vi "Read Output.vi"(8 "error in":errorcluster, 11 "2230G in":refnum<class "2230G.lvclass">) -> (0 "error out":errorcluster, 2 "Output":bool, 3 "2230G out":refnum<class "2230G.lvclass">)   [LabVIEW 2018, in "2230G.lvlib" / "2230G.lvclass"]
uses:
  2230G.lvclass
  <vilib>/regexp/Match Regular Expression.xnode
  PPLs/Power Supply/Parent/Power_Supply.lvlibp/Power Supply.lvclass
  <instrlib>/Keithley KE22xx Series/Keithley KE22xx Series.lvlib
  C:/Projects/LabVIEW/PPLs/Power Supply/Parent/Power_Supply.lvlibp/Power Supply.lvclass
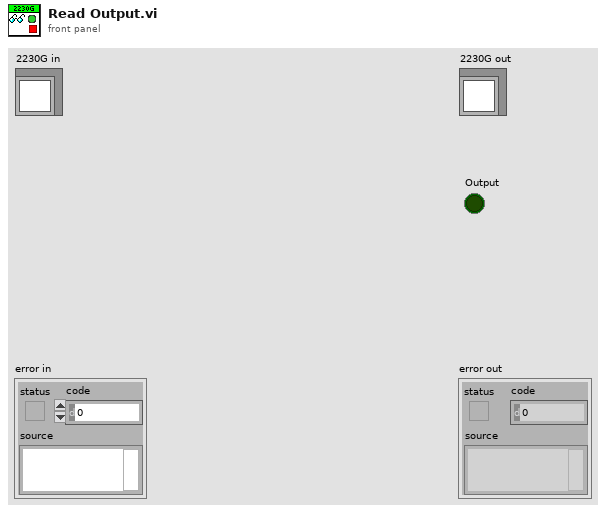
[diagram p1: front panel]
types:
  T1 = typedef "Power_Supply.lvlibp/Channel List.ctl" = enum16{"Channel 1", "Channel 2", "Channel 3", "Channel 4"}
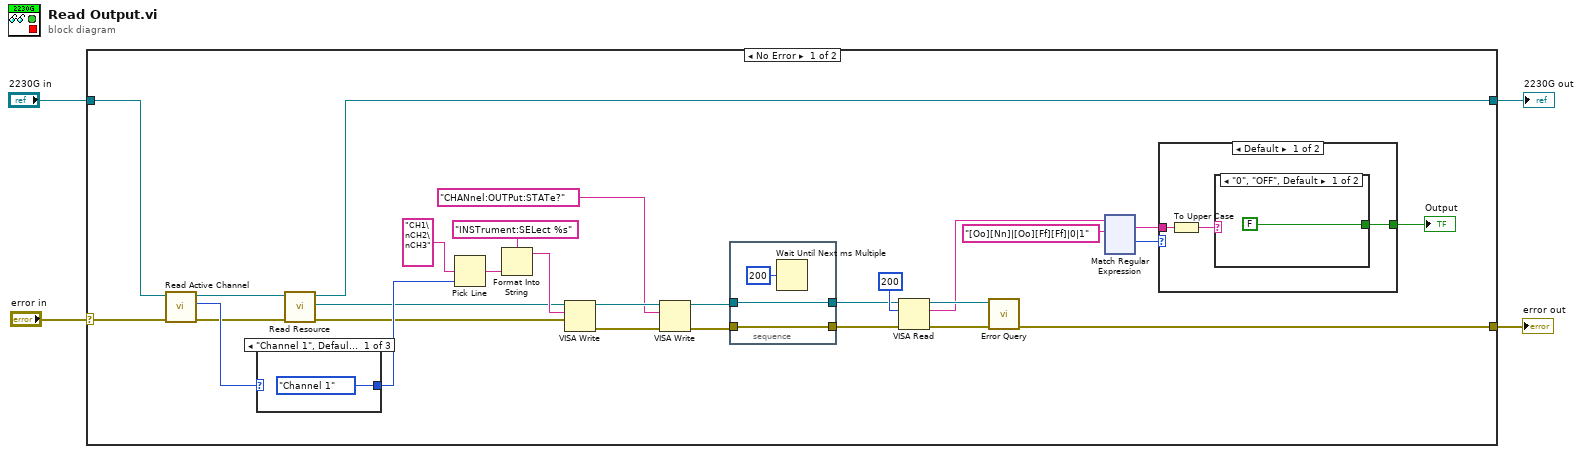
[diagram p0: block diagram]
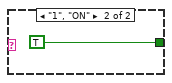
[diagram p2: hidden frame]
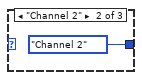
[diagram p4: hidden frame]
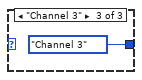
[diagram p5: hidden frame]
diagram:
  n1 = case shown="No Error" "error in" {
    selector: "error in" -> [w5 w160]
    tunnel: [w11 w160] -> w2
    tunnel: [w29 w159] -> w3
    tunnel: "2230G in" -> [w33 w159]
    frame No Error {
      n2 = call "Read Active Channel.vi"("error in (no error)"=w5, "Power Supply in"=w33) -> ("error out"=w30:errorcluster, "Active Channel"=w31:T1, "Power Supply out"=w32:refnum<class "2230G.lvclass">)  [unwired: 7 in]
      n3 = case shown="\"Channel 1\", Default" w31 {
        tunnel: [enum16{"Channel 1", "Channel 2", "Channel 3"}."Channel 1" ("Channel Select") enum16{"Channel 1", "Channel 2", "Channel 3"}."Channel 2" ("Channel Select") enum16{"Channel 1", "Channel 2", "Channel 3"}."Channel 3" ("Channel Select")] -> w24
        frame "Channel 1", Default {
        }
        frame "Channel 2" {
        }
        frame "Channel 3" {
        }
      }
      n4 = call "Read Resource.vi"("error in"=w30, "Power Supply in"=w32) -> ("error out"=w22:errorcluster, "Resource"=w23:refnum<visa-resource-name>, "Power Supply out"=w29:refnum<class "2230G.lvclass">)  [unwired: 7 in]
      n5 = Pick Line(multi-line string="CH1\nCH2\nCH3", line index=w24) -> (output string=w27:string)  [unwired: 1 in]
      n6 = Format Into String(format string="INSTrument:SELect %s", w27) -> (resulting string=w25:string)  [unwired: 2 in, 1 out]
      n7 = VISA Write(VISA resource name=w23, write buffer=w25, error in (no error)=w22) -> (VISA resource name out=w21:refnum<visa-resource-name>, error out=w20:errorcluster)  [unwired: 1 out]
      n8 = VISA Write(VISA resource name=w21, write buffer="CHANnel:OUTPut:STATe?", error in (no error)=w20) -> (VISA resource name out=w12:refnum<visa-resource-name>, error out=w13:errorcluster)  [unwired: 1 out]
      n9 = stacked-sequence {
        tunnel: [w155] -> w15
        tunnel: w12 -> [w155]
        tunnel: w13 -> [w154]
        tunnel: [w154] -> w14
        frame #0 {
          n10 = Wait Until Next ms Multiple(millisecond multiple=u32 200 ("Programmable Delay in ms")) -> ()  [unwired: 1 out]
        }
      }
      n11 = VISA Read(VISA resource name=w15, byte count=u32 200, error in (no error)=w14) -> (VISA resource name out=w18:refnum<visa-resource-name>, read buffer=w10:string, error out=w17:errorcluster)  [unwired: 1 out]
      n12 = call <instrlib>:"Error Query.vi"("error in (no error)"=w17, "VISA resource name"=w18) -> ("error out"=w11:errorcluster)  [unwired: 6 in, 3 out]
      n13 = xnode "Match Regular Expression"("input string"=w10, "regular expression"="[Oo][Nn]|[Oo][Ff][Ff]|0|1") -> ("whole match"=w7:string, "offset past match"=w8:i32)  [unwired: 4 in, 3 out]
      n14 = case shown="Default" w8 {
        tunnel: w7 -> [w36 _]
        tunnel: [w34 _] -> w6
        frame Default {
          n15 = To Upper Case(1:w36) -> (0:w35:string)
          n16 = case shown="\"0\", \"OFF\", Default" w35 {
            tunnel: [FALSE TRUE] -> w34
            frame "0", "OFF", Default {
            }
            frame "1", "ON" {
            }
          }
        }
        frame -1 {
        }
      }
      "Output" <- w6
    }
    frame Error {
    }
  }
  "error out" <- w2
  "2230G out" <- w3
